vi "PC_DCG to DECM HW timed DAQ1 to DAQ2.vi"() -> ()   [LabVIEW 2021]
uses:
  Digital Edge Count Measurement/Typedefs/Measurement Settings.ctl
  Digital Edge Count Measurement/Typedefs/Wait Type.ctl
  Digital Edge Count Measurement/Typedefs/Timer - Trigger Settings.ctl
  Digital Clock Generation/Typedefs/Digital Clock Settings.ctl
  Digital Clock Generation/Typedefs/Actual Clock Settings.ctl
  Common/Typedefs/Execution Options - Measure.ctl
  Digital Edge Count Measurement/DAQ_Digital Edge Count Measurement.lvlib
  Digital Clock Generation/DAQ_Digital Clock Generation.lvlib
panel:
  out "Actual Clock Settings":T1={"Frequency (Hz)"=1000.0, "Duty Cycle (%)"=50.0, "Generation Time (s)"=1.0} {"Duty Cycle (%)" format="%#.2p"; "Frequency (Hz)" format="%.6p"; "Generation Time (s)" format="%.2p"}
  in  "Digital Clock Settings":T2={"Frequency (Hz)"=1000.0, "Duty Cycle(%)"=50.0, "Generation Time (s)"=1.0} {"Duty Cycle(%)" format="%#.2p"; "Frequency (Hz)" format="%.6p"; "Generation Time (s)" format="%.2p"}
  out "Edge Counts":u32=1000
  out "error out":errorcluster
  in  "Timer - Trigger Settings":T3={"Trigger Type"=enum."Digital Start", "Digital Start Trigger Source"="/Dev2/PFI0", "Digital Start Trigger Edge"=10280} {"Digital Start Trigger Edge" items=["Rising"=10280, "Falling"=10171]}
  in  "Counter Settings":T4={"Active Edge"=10171, "Duration (s)"=1.0, "Wait Type"=enum."Hardware Timed"} {"Duration (s)" format="%.2p"; "Active Edge" items=["Rising"=10280, "Falling"=10171]}
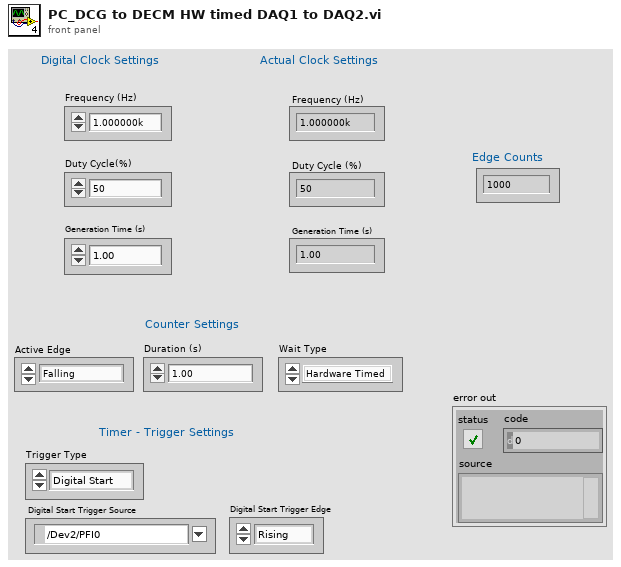
[diagram p1: front panel]
types:
  T1 = typedef "DAQ_Digital Clock Generation.lvlib/Actual Clock Settings.ctl" = cluster{"Frequency (Hz)":dbl, "Duty Cycle (%)":dbl, "Generation Time (s)":dbl}
  T2 = typedef "DAQ_Digital Clock Generation.lvlib/Digital Clock Settings.ctl" = cluster{"Frequency (Hz)":dbl, "Duty Cycle(%)":dbl, "Generation Time (s)":dbl}
  T3 = typedef "DAQ_Digital Edge Count Measurement.lvlib/Timer - Trigger Settings.ctl" = cluster{"Trigger Type":enum16{"No Trigger", "Digital Start"}, "Digital Start Trigger Source":tag, "Digital Start Trigger Edge":i32}
  T4 = typedef "DAQ_Digital Edge Count Measurement.lvlib/Measurement Settings.ctl" = cluster{"Active Edge":i32, "Duration (s)":dbl, "Wait Type":T5}
  T5 = typedef "DAQ_Digital Edge Count Measurement.lvlib/Wait Type.ctl" = enum16{"Hardware Timed", "Software Timed"}
  T6 = typedef "Execution Options - Measure.ctl" = enum16{"Configure & Measure", "Configure only", "Measure only"}
  T7 = typedef "DAQ_Digital Edge Count Measurement.lvlib/DAQmx Tasks.ctl" = cluster{"Counter DAQmx Task":refnum<k21>, "Timer DAQmx Task":refnum<k21>}
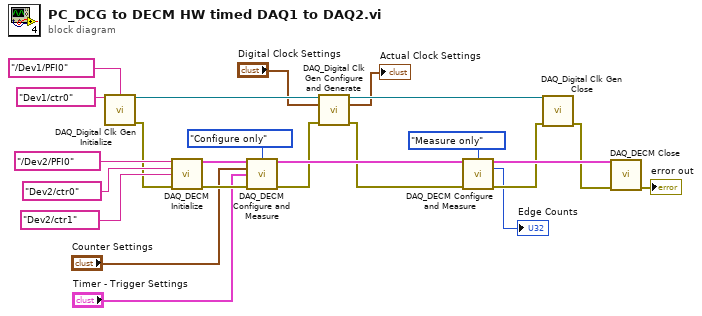
[diagram p0: block diagram]
diagram:
  n1 = call "DAQ_Digital Clk Gen Initialize.vi"("Physical Channel (Counter)"=tag "Dev1/ctr0", "Output Terminal"=tag "/Dev1/PFI0") -> ("DAQmx Task Out"=w24:refnum<k21>, "error out"=w17:errorcluster)  [unwired: 12 in]
  n2 = call "DAQ_DECM Initialize.vi"("Input Terminal"=tag "/Dev2/PFI0", "Counter - Edge Counting"=tag "Dev2/ctr0", "Counter - Timer"=tag "Dev2/ctr1", "error in"=w17) -> ("DAQmx Tasks"=w15:T7, "error out"=w16:errorcluster)  [unwired: 10 in]
  n3 = call "DAQ_DECM Configure and Measure.vi"("DAQmx Tasks In"=w15, "Execution Option"=Execution_Options_-_Measure."Configure only", "Counter Settings"="Counter Settings", "Timer - Trigger Settings"="Timer - Trigger Settings", "error in"=w16) -> ("DAQmx Tasks Out"=w14:T7, "error out"=w9:errorcluster)  [unwired: 8 in, 1 out]
  n4 = call "DAQ_Digital Clk Gen Configure and Generate.vi"("DAQmx Task In"=w24, "Digital Clock Settings"="Digital Clock Settings", "error in"=w9) -> ("DAQmx Task Out"=w23:refnum<k21>, "Actual Clock Settings"=→"Actual Clock Settings":T1, "error out"=w10:errorcluster)  [unwired: 10 in]
  n5 = call "DAQ_DECM Configure and Measure.vi"("DAQmx Tasks In"=w14, "Execution Option"=Execution_Options_-_Measure."Measure only", "error in"=w10) -> ("DAQmx Tasks Out"=w13:T7, "Edge Counts"=→"Edge Counts":u32, "error out"=w11:errorcluster)  [unwired: 10 in]
  n6 = call "DAQ_Digital Clk Gen Close.vi"("DAQmx Task In"=w23, "error in"=w11) -> ("error out"=w12:errorcluster)  [unwired: 13 in]
  n7 = call "DAQ_DECM Close.vi"("DAQmx Tasks"=w13, "error in"=w12) -> ("error out"=→"error out":errorcluster)  [unwired: 13 in]
